vi "sub_manipulator_command.vi"(8 "error in":errorcluster, 9 "Cycles":i16[](array[numeric]), 10 "I2C interface":T1) -> (0 "error out":errorcluster)   [LabVIEW 2014]
uses:
  i2c_interface.ctl
  fpga_reference.ctl
  <vilib>/Utility/error.llb/Error Cluster From Error Code.vi
  <vilib>/rvi/errors/niLvFpgaAdjustHostInterfaceError.vi
  <vilib>/rvi/interface/nirviMethod/nirviMethod.xnode
  FPGA Bitfiles/i2cmuxdemux.lvbitx
  <vilib>/FPGAPlugInAG/PCIe-7842R/niLvFpga_WriteFifo_PCIe-7842R.vi
  <vilib>/rvi/errors/niLvFpgaMergeErrorWithErrorCode.vi
panel:
  in  "Sequence number":u8
  # "The main part of marshalling data to send to FPGA for the write-all-axes squiggle motor command interface."
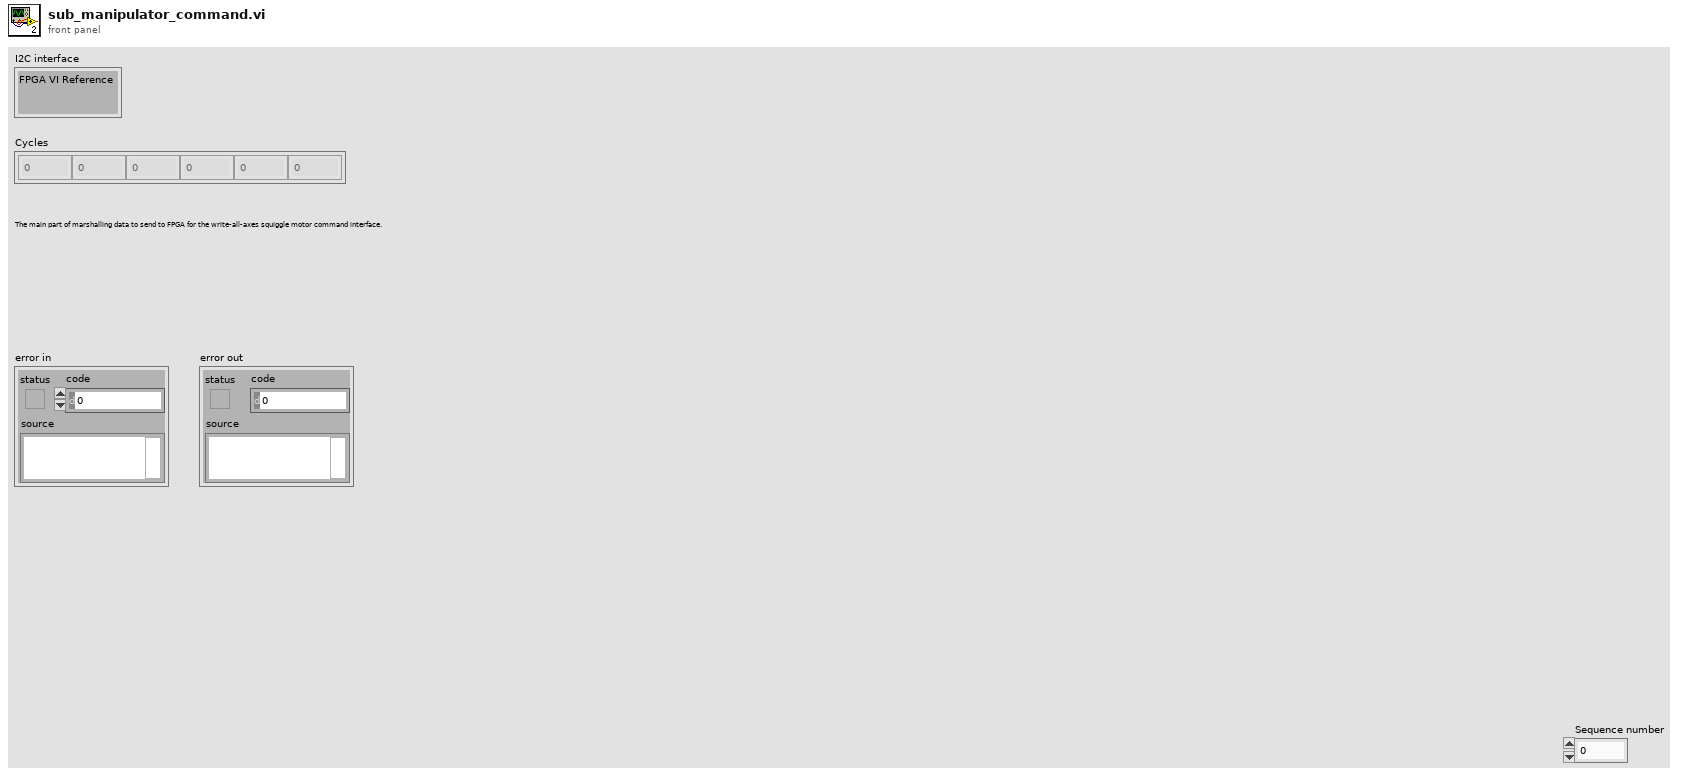
[diagram p1: front panel]
types:
  T1 = typedef "i2c_interface.ctl" = cluster{"FPGA VI Reference":T2}
  T2 = typedef "fpga_reference.ctl" = refnum<k20>
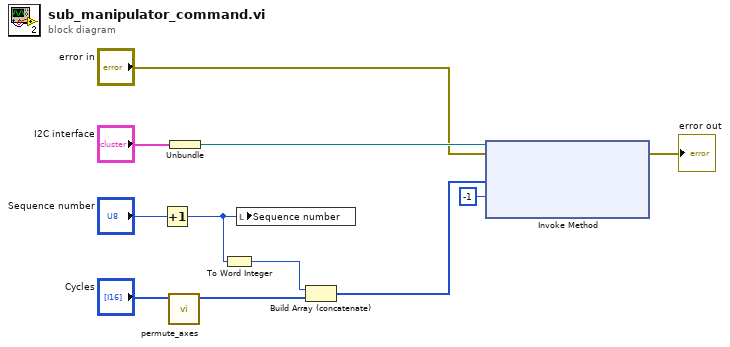
[diagram p0: block diagram]
diagram:
  n1 = Increment(x="Sequence number") -> (x+1=w8:u8)
  n2 = call "permute_axes.vi"("Pulse count"="Cycles") -> ("Result"=w3:i16[])  [unwired: 10 in]
  n3 = Unbundle("I2C interface") -> ("FPGA VI Reference"=w7:T2)
  n4 = To Word Integer(number=w8) -> (16bit integer=w6:i16)
  n5 = local write "Sequence number"(w8) -> ()
  n6 = Build Array (concatenate)(w6, w3) -> (w2:i16[])
  n7 = xnode "Invoke Method"("FPGA VI Reference In"=w7, "error in"="error in", "Data"=w2, "Timeout (ms)"=-1) -> ("error out"=→"error out":errorcluster)  [unwired: 2 out]
